vi "RemoveGjoints.vi"(1 "remaining 2":string) -> (0 "remaining":string)   [LabVIEW 2012]
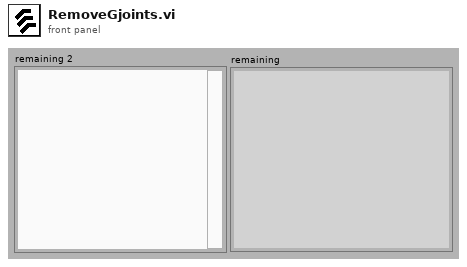
[diagram p1: front panel]
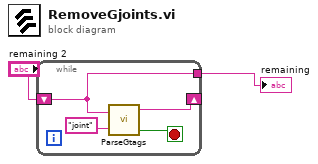
[diagram p0: block diagram]
diagram:
  n1 = while {
    shift-right: [w4] -> _
    shift-left: "remaining 2" -> [w3]
    tunnel: [w3] -> w2
    stop <- w5 stop-if-true
    n2 = call <userlib>:"ParseGtags.vi"("tag"="joint", "urdf in"=w3) -> ("not found"=w5:bool, "urdf out"=w4:string)  [unwired: 2 out]
  }
  "remaining" <- w2
